vi "Reset AI Tasks.vi"(8 "error in":errorcluster, 11 "CRDS in":refnum<class "CRDS.lvclass">) -> (0 "error out":errorcluster, 3 "CRDS out":refnum<class "CRDS.lvclass">)   [LabVIEW 2011]
uses:
  CRDS.lvclass
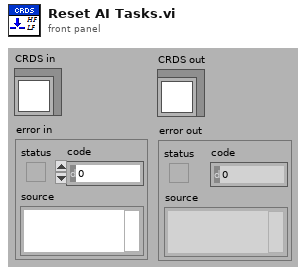
[diagram p1: front panel]
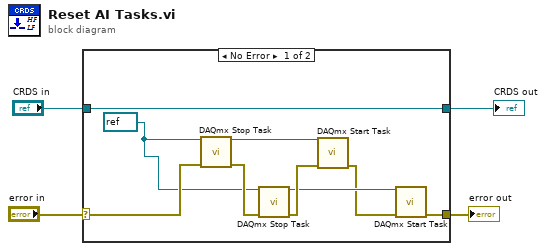
[diagram p0: block diagram]
diagram:
  n1 = case shown="No Error" "error in" {
    selector: "error in" -> [w12 w15]
    tunnel: [w6 w15] -> w3
    tunnel: [w13 w14] -> w1
    tunnel: "CRDS in" -> [w13 w14]
    frame No Error {
      w5 = refnum<k21> refnum ("task/channels in")
      n2 = call <vilib>:"DAQmx Stop Task.vi"("task/channels in"=w5, "error in"=w12) -> ("task out"=w10:refnum<k21>, "error out"=w11:errorcluster)  [unwired: 12 in]
      n3 = call <vilib>:"DAQmx Stop Task.vi"("task/channels in"=w5, "error in"=w11) -> ("task out"=w8:refnum<k21>, "error out"=w9:errorcluster)  [unwired: 12 in]
      n4 = call <vilib>:"DAQmx Start Task.vi"("task/channels in"=w10, "error in"=w9) -> ("error out"=w7:errorcluster)  [unwired: 12 in, 1 out]
      n5 = call <vilib>:"DAQmx Start Task.vi"("task/channels in"=w8, "error in"=w7) -> ("error out"=w6:errorcluster)  [unwired: 12 in, 1 out]
    }
    frame Error {
    }
  }
  "error out" <- w3
  "CRDS out" <- w1
